vi "ELVIS III v1.0 Unreserve AO Continuous.vi"(8 "error in (no error)":errorcluster, 11 "AO (Continuous) Channels List":T1 caption="AI (Continuous) Channels List") -> (0 "error out":errorcluster)   [LabVIEW 2021]
uses:
  <vilib>/myRIO/Common/Instrument Driver Framework/ELVIS III v1.0/AO Continuous/typedefs/AO Continuous Channels List.ctl
  <vilib>/myRIO/Common/Instrument Driver Framework/ELVIS III v1.0/AO Continuous/typedefs/ELVIS III v1.0 AO Continuous Channels Enum.ctl
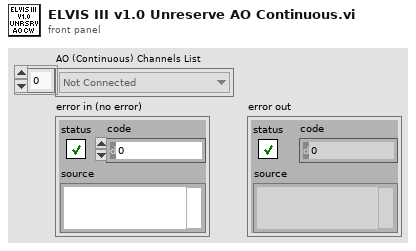
[diagram p1: front panel]
types:
  T1 = typedef "AO Continuous Channels List.ctl" = T2[]
  T2 = typedef "ELVIS III v1.0 AO Continuous Channels Enum.ctl" = enum16{"Not Connected", "A/AO0 (Continuous)", "A/AO1 (Continuous)", "B/AO0 (Continuous)", "B/AO1 (Continuous)"}
  T3 = typedef "ELVIS III v1.0 Channel Reservation List.ctl" = T4[]
  T4 = typedef "ELVIS III v1.0 Channel Reservation Info.ctl" = cluster{"Channel Name":string, "Connector":T5, "MutexIDs":u32[]}
  T5 = typedef "ELVIS III v1.0 Connector List.ctl" = enum32{"None", "ConnectorA", "ConnectorB"}
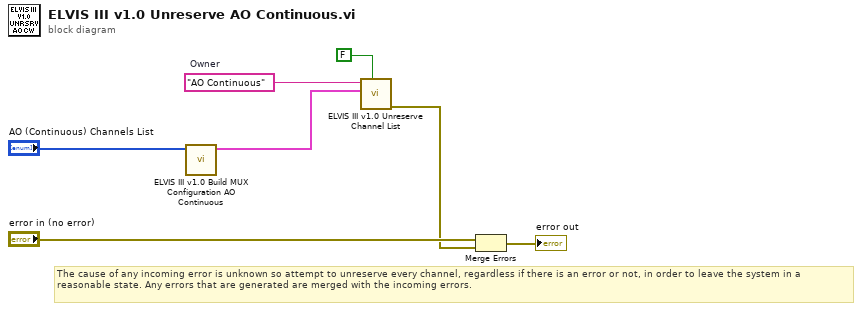
[diagram p0: block diagram]
diagram:
  w4 = "AO Continuous"  # Owner
  # "The cause of any incoming error is unknown so attempt to unreserve every channel, regardless if there is an error or not, in order to leave the system in a reasonable state. Any errors that are generated are merged with the incoming errors."
  n1 = call <vilib>:"ELVIS III v1.0 Build MUX Configuration AO Continuous.vi"("AO (Continuous) Channels List"="AO (Continuous) Channels List") -> ("Channel Reservation Info"=w5:T3)  [unwired: 10 in]
  n2 = call <vilib>:"ELVIS III v1.0 Unreserve Channel List.vi"("Allow multiple opens?"=FALSE, "Channel Reservation List"=w5, "Owner"=w4) -> ("error out"=w3:errorcluster)  [unwired: 8 in]
  n3 = Merge Errors("error in (no error)", w3) -> (→"error out":errorcluster)
